vi "SeeTheThing.vi"(0 "Image In":T2, 7 "error in":errorcluster) -> (20 "Image Out":T2, 21 "Matches (Color Location 1)":T1(array[cluster]) {"Bounding Box"."y" format="%.2f"; "Bounding Box"."x" format="%.2f"; "Position"."y" format="%.2f"; "Position"."x" format="%.2f"; "Score" format="%.2f"; "Scale" format="%.2f"; "Angle" format="%.2f"}, 22 "Matches (calibrated) (Color Location 1)":T1(array[cluster]) {"Bounding Box"."y" format="%.2f"; "Bounding Box"."x" format="%.2f"; "Position"."y" format="%.2f"; "Position"."x" format="%.2f"; "Score" format="%.2f"; "Scale" format="%.2f"; "Angle" format="%.2f"}, 23 "Number of Matches (Color Location 1)":i32, 27 "error out":errorcluster)   [LabVIEW 2016]
uses:
  <vilib>/vision/Image Controls.llb/IMAQ Image.ctl
  <vilib>/vision/NI_Vision_Development_Module.lvlib
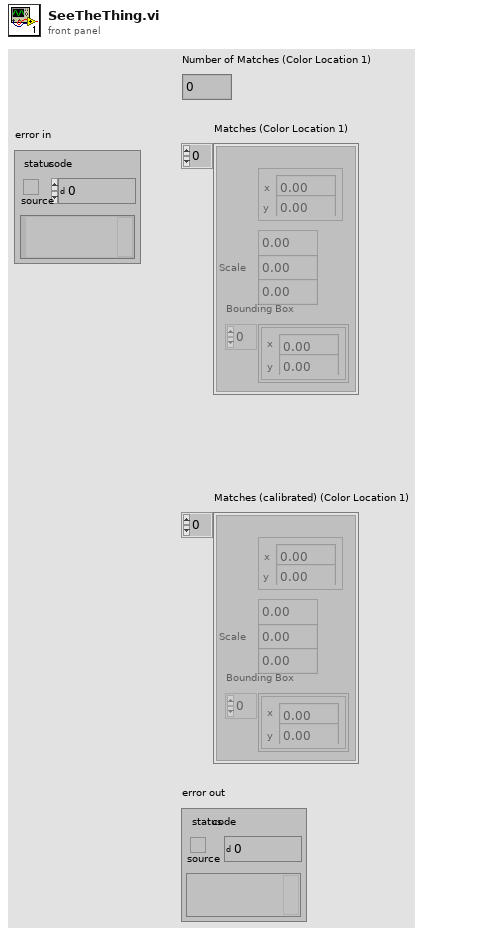
[diagram p1: front panel]
types:
  T1 = cluster{"Position":cluster{"x":sgl, "y":sgl}, "Angle":sgl, "Scale":sgl, "Score":sgl, "Bounding Box":cluster{"x":sgl, "y":sgl}[]}[]
  T2 = typedef "IMAQ Image.ctl" = refnum<image>
  T3 = typedef "Image Type" = u32
  T4 = cluster{"Global Rectangle":i32[], "Contours":cluster{"ID":enum32{"External", "Internal"}, "Type":u32, "Coordinates":i32[]}[]}
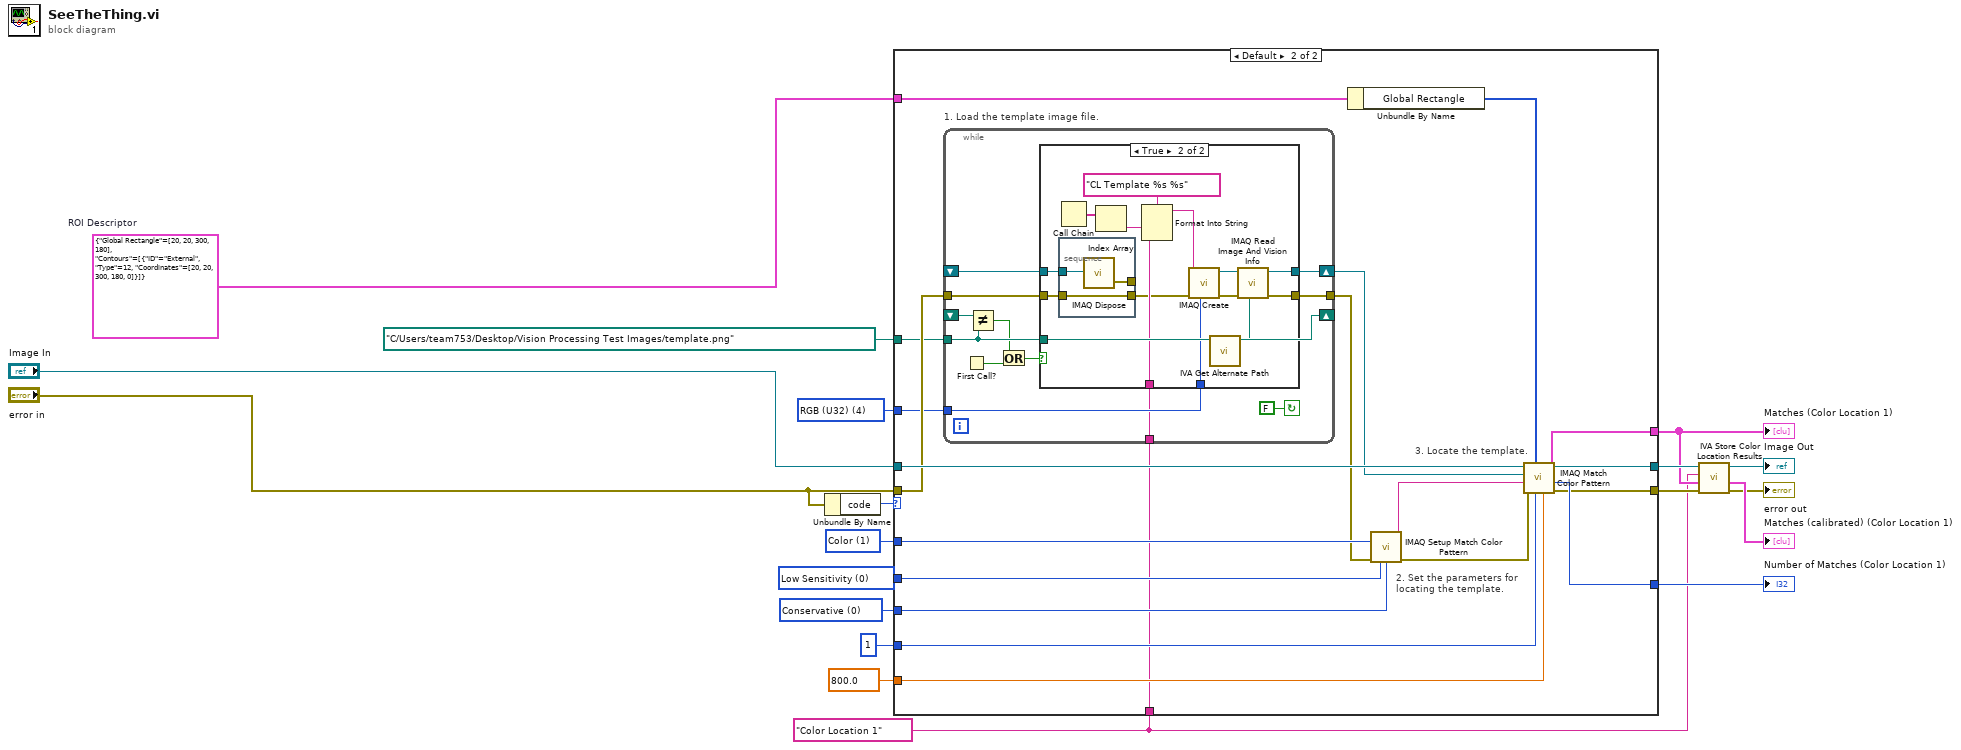
[diagram p0: block diagram]
diagram:
  w1 = "Color Location 1" ("Step Name")
  w11 = T3 4 items=["Grayscale (U8)", "Grayscale (I16)", "Grayscale (SGL)", "Complex (CSG)", "RGB (U32)", "HSL (U32)", "RGB (U64)"] ("Image Type")
  w13 = u32 0 items=["Conservative", "Balance", "Aggressive", "Very Aggressive"] ("Search Strategy")
  w14 = u32 0 items=["Low Sensitivity", "Medium Sensitivity", "High Sensitivity"] ("Color Sensitivity")
  w15 = u32 1 items=["Color and Shape", "Color", "Shape"] ("Match Feature Mode")
  w10 = T4 {"Global Rectangle"=[20, 20, 300, 180], "Contours"=[{"ID"=enum."External", "Type"=12, "Coordinates"=[20, 20, 300, 180, 0]}]}  # ROI Descriptor
  n1 = Unbundle By Name("error in") -> ("code"=w8:i32)
  n2 = case shown="Default" w8 {
    tunnel: sgl 800.0 ("Minimum Match Score") -> [_ w39]
    tunnel: 1 ("Number of Matches Requested") -> [_ w38]
    tunnel: [_ w37] -> w16
    tunnel: w15 -> [_ w36]
    tunnel: w14 -> [_ w35]
    tunnel: w13 -> [_ w34]
    tunnel: path "C:/Users/team753/Desktop/Vision Processing Test Images/template.png" ("File Path") -> [_ w26]
    tunnel: w11 -> [_ w25]
    tunnel: "error in" -> [_ w27]
    tunnel: w10 -> [_ w31]
    tunnel: [_ w29] -> w2
    tunnel: "Image In" -> [w20 w28]
    tunnel: [w20 w28] -> w3
    tunnel: [_ w22] -> w5
    tunnel: w1 -> [_ w21]
    frame -1074396199, -1074396198 {
      # "Discard Coordinate System Error"
    }
    frame Default {
      # "3. Locate the template."
      # "2. Set the parameters for\nlocating the template."
      n3 = while "1. Load the template image file." {
        shift-right: [w51] -> w24
        shift-left: _ -> [w50]
        tunnel: [w48] -> w23
        tunnel: w27 -> [w47]
        tunnel: w26 -> [w43]
        tunnel: w25 -> [w46]
        tunnel: w21 -> [w45]
        shift-right: [w43] -> _
        shift-left: _ -> [w44]
        stop <- FALSE continue-if-true
        n4 = First Call?() -> (First Call?: T/F=w42:bool)
        n5 = Not Equal?(x=w44, y=w43) -> (x != y?=w41:bool)
        n6 = Or(x=w41, y=w42) -> (x .or. y?=w40:bool)
        n7 = case shown="True" w40 {
          tunnel: [w53 w66] -> w51
          tunnel: w50 -> [w53 w58]
          tunnel: [w52 w63] -> w48
          tunnel: w47 -> [w52 w57]
          tunnel: w46 -> [_ w62]
          tunnel: w45 -> [_ w59]
          tunnel: w43 -> [_ w55]
          frame False {
          }
          frame True {
            n8 = Call Chain() -> (call chain=w61:string[])
            n9 = stacked-sequence {
              tunnel: w58 -> [w71]
              tunnel: w57 -> [w70]
              tunnel: [w70] -> w56
              tunnel: [w69] -> _
              frame #0 {
                n10 = call "IMAQ Dispose"("Image"=w71) -> ("error out"=w69:errorcluster)  [unwired: 2 in, 3 out]
              }
            }
            n11 = Index Array(array=w61) -> (element=w60:string)  [unwired: 1 in]
            n12 = Format Into String(format string="CL Template %s %s" ("Image Name"), w60, w59) -> (resulting string=w68:string)  [unwired: 2 in, 1 out]
            n13 = call "IMAQ Create"("Image Name"=w68, "Image Type"=w62, "error in (no error)"=w56) -> ("New Image"=w65:T2, "error out"=w64:errorcluster)  [unwired: 1 in, 1 out]
            n14 = call <vilib>:"IVA Get Alternate Path.vi"("Path In"=w55) -> ("Path Out"=w54:path)  [unwired: 10 out]
            n15 = call "IMAQ Read Image And Vision Info"("File Path"=w54, "error in (no error)"=w64, "Image"=w65) -> ("error out"=w63:errorcluster, "Image Out"=w66:T2)  [unwired: 1 in, 6 out]
          }
        }
      }
      n16 = Unbundle By Name(w31) -> ("Global Rectangle"=w30:i32[])
      n17 = call "IMAQ Setup Match Color Pattern"("Match Feature Mode"=w36, "error in (no error)"=w23, "Color Sensitivity"=w35, "Search Strategy"=w34) -> ("Match Color Pattern Setup Data"=w33:string, "error out"=w32:errorcluster)  [unwired: 5 in, 5 out]
      n18 = call "IMAQ Match Color Pattern"("Minimum Match Score"=w39, "Number of Matches Requested"=w38, "Optional Rectangle"=w30, "error in (no error)"=w32, "Match Color Pattern Setup Data"=w33, "Template Image"=w24, "Image"=w28) -> ("error out"=w22:errorcluster, "Number of Matches"=w37:i32, "Matches"=w29:T1)  [unwired: 2 out]
    }
  }
  "Number of Matches (Color Location 1)" <- w16
  "Matches (Color Location 1)" <- w2
  n19 = call <vilib>:"IVA Store Color Location Results.vi"("error in (no error)"=w5, "Matches"=w2, "Step Name"=w1, "Image in"=w3) -> ("error out"=→"error out":errorcluster, "Calibrated Matches"=→"Matches (calibrated) (Color Location 1)":T1, "Image dup"=→"Image Out":T2)  [unwired: 5 out]
